vi "JKI SM Editor - Pre-Build Custom Action.vi"(10 "Variant":variant) -> (0 "error out":errorcluster)   [LabVIEW 2020]
uses:
  <userlib>/_OpenG.lib/file/file.llb/openg_file.lvlib
  <vilib>/JKI/VIPM API/VIPM API_vipm_api.lvlib
  <userlib>/_OpenG.lib/error/error.llb/openg_error.lvlib
  <userlib>/_OpenG.lib/file/file.llb/Compare Two Paths - Scalar__ogtk.vi
  <vilib>/JKI/VIPM API/Apply VIPC File_vipm_api.vi
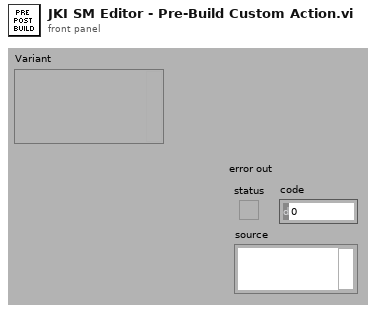
[diagram p1: front panel]
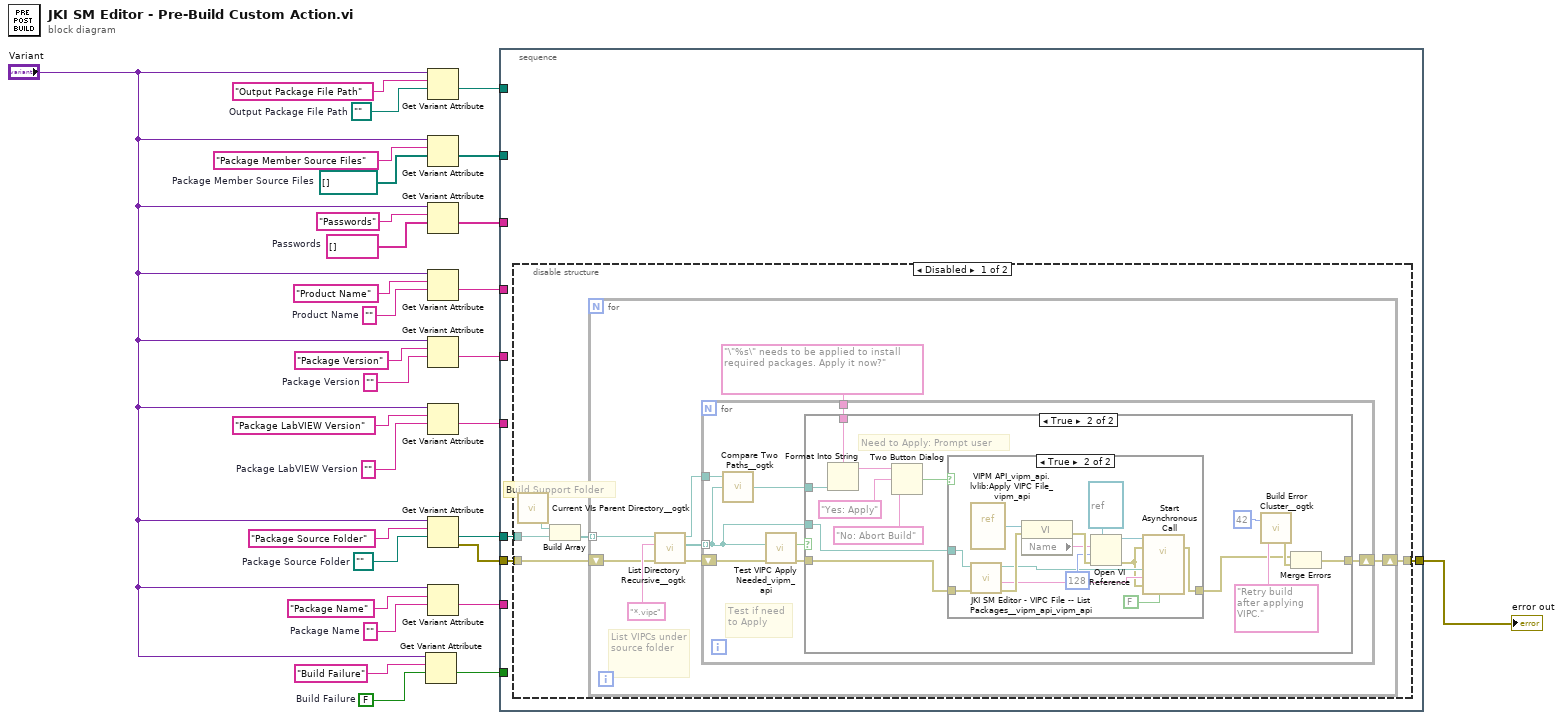
[diagram p0: block diagram]
diagram:
  w5 = FALSE  # Build Failure
  w15 = path ""  # Package Source Folder
  w16 = ""  # Package Name
  w19 = ""  # Package LabVIEW Version
  w21 = ""  # Package Version
  w23 = ""  # Product Name
  w25 = string[] []  # Passwords
  w27 = path[] []  # Package Member Source Files
  w29 = path ""  # Output Package File Path
  n1 = Get Variant Attribute(Variant="Variant", name="Build Failure", default value (empty Variant)=w5) -> (value=w3:bool)  [unwired: 1 in, 3 out]
  n2 = Get Variant Attribute(Variant="Variant", name="Output Package File Path", default value (empty Variant)=w29) -> (value=w14:path)  [unwired: 1 in, 3 out]
  n3 = Get Variant Attribute(Variant="Variant", name="Package Member Source Files", default value (empty Variant)=w27) -> (value=w13:path[])  [unwired: 1 in, 3 out]
  n4 = Get Variant Attribute(Variant="Variant", name="Passwords", default value (empty Variant)=w25) -> (value=w12:string[])  [unwired: 1 in, 3 out]
  n5 = Get Variant Attribute(Variant="Variant", name="Product Name", default value (empty Variant)=w23) -> (value=w11:string)  [unwired: 1 in, 3 out]
  n6 = Get Variant Attribute(Variant="Variant", name="Package Version", default value (empty Variant)=w21) -> (value=w10:string)  [unwired: 1 in, 3 out]
  n7 = Get Variant Attribute(Variant="Variant", name="Package LabVIEW Version", default value (empty Variant)=w19) -> (value=w9:string)  [unwired: 1 in, 3 out]
  n8 = Get Variant Attribute(Variant="Variant", name="Package Source Folder", default value (empty Variant)=w15) -> (value=w8:path, error out=w2:errorcluster)  [unwired: 1 in, 2 out]
  n9 = Get Variant Attribute(Variant="Variant", name="Package Name", default value (empty Variant)=w16) -> (value=w7:string)  [unwired: 1 in, 3 out]
  n10 = stacked-sequence {
    tunnel: w14 -> [_]
    tunnel: w13 -> [_]
    tunnel: w12 -> [_]
    tunnel: w11 -> [_]
    tunnel: w10 -> [_]
    tunnel: w9 -> [_]
    tunnel: w8 -> [w33]
    tunnel: w7 -> [_]
    tunnel: w3 -> [_]
    tunnel: w2 -> [w32]
    tunnel: [w31] -> w1
    frame #0 {
      n11 = disable-structure shown="Disabled" {
        disable-tunnel: w33 -> [w38 _]
        disable-tunnel: w32 -> [w37 _]
        disable-tunnel: [w36 _] -> w31
        frame Disabled {
          # "Build Support Folder"
          n12 = call <userlib>:"Current VIs Parent Directory__ogtk.vi"() -> ("Parent Directory (+ Relative)"=w34:path)  [unwired: 5 in]
          n13 = Build Array(w34, w38) -> (w35:path[])
          n14 = for {
            tunnel: w35 -> [w45] mode=indexing
            shift-right: [w39] -> w36
            shift-left: w37 -> [w44]
            # "List VIPCs under source folder"
            n15 = call <userlib>:"List Directory Recursive__ogtk.vi"("error in (no error)"=w44, "pattern"="*.vipc", "Path"=w45) -> ("error out"=w43:errorcluster, "file paths"=w42:path[], "dup Path"=w41:path)  [unwired: 5 in, 1 out]
            n16 = for {
              tunnel: w42 -> [w47] mode=indexing
              shift-right: [w48] -> w39
              shift-left: w43 -> [w54]
              tunnel: w41 -> [w51]
              tunnel: "\"%s\" needs to be applied to install required packages. Apply it now?" ("message") -> [w49]
              # "Test if need to Apply"
              n17 = call-poly <userlib>:"Compare Two Paths__ogtk.vi"("path2"=w47, "path1"=w51) -> ("relative path from 1 to 2"=w50:path)  [unwired: 1 in, 2 out]
              n18 = call <vilib>:"Test VIPC Apply Needed_vipm_api.vi"("error in (no error)"=w54, "VIPC File Path"=w47) -> ("error out"=w52:errorcluster, "Need to Apply?"=w53:bool)  [unwired: 7 in, 1 out]
              n19 = case shown="True" w53 {
                tunnel: w52 -> [w55 w58]
                tunnel: w50 -> [_ w68]
                tunnel: w49 -> [_ w67]
                tunnel: w47 -> [_ w57]
                tunnel: [w55 w63] -> w48
                frame False {
                  # "No need to apply. Proceed."
                }
                frame True {
                  # "Need to Apply: Prompt user"
                  n20 = Format Into String(format string=w67, w68) -> (resulting string=w66:string)  [unwired: 2 in, 1 out]
                  n21 = Two Button Dialog(message=w66, 1:"No: Abort Build" ("F button name (\"Cancel\")"), 2:"Yes: Apply" ("T button name (\"OK\")")) -> (T button?=w59:bool)
                  n22 = case shown="True" w59 {
                    tunnel: w58 -> [w69 w77]
                    tunnel: w57 -> [_ w75]
                    tunnel: [w69 w70] -> w56
                    frame False {
                    }
                    frame True {
                      n23 = vi-ref "VIPM API_vipm_api.lvlib:Apply VIPC File_vipm_api.vi"() -> (w80:refnum<vi>)
                      n24 = call "JKI SM Editor - VIPC File -- List Packages__vipm_api_vipm_api.vi"("error in (no error)"=w77, "VIPC File Path"=w75) -> ("error out"=w76:errorcluster, "VIPC LabVIEW Version"=w74:string, "VIPC File Path (dup)"=w73:path)  [unwired: 6 in, 1 out]
                      n25 = property class="VI"(reference=w80, error in=w76) -> (error out=w83:errorcluster, "Name"=w81:string)  [unwired: 1 out]
                      n26 = Open VI Reference(type specifier VI Refnum (for type only)=refnum<vi> refnum, vi path=w81, options=128, error in (no error)=w83) -> (vi reference=w78:refnum<vi>, error out=w71:errorcluster)  [unwired: 2 in]
                      n27 = call-by-ref "Start Asynchronous Call"(reference=w78, error in=w71, "quiet? (T)"=FALSE, 8:"error in (no error)"=w71, "LabVIEW Version"=w74, "VIPC File"=w73) -> (error out=w70:errorcluster)  [unwired: 7 in, 2 out]
                    }
                  }
                  n28 = call <userlib>:"Build Error Cluster__ogtk.vi"("String to Prepend to source (\"\")"="Retry build after applying VIPC." ("String to Prepend to source (\"\")"), "code"=42) -> ("error out"=w61:errorcluster)
                  n29 = Merge Errors(w56, w61) -> (w63:errorcluster)
                }
              }
            }
          }
        }
        frame Enabled {
        }
      }
    }
  }
  "error out" <- w1
